vi "target.vi"   [LabVIEW 2020]
uses:
  <vilib>/rvi/interface/RandomDataEmulation/niFpgaRandomDataHandleErrors.vi
  matrix_matrix_multiply_FXP_16_4.vi
  <vilib>/rvi/DataTransferAndStorage/Container/XNode/niFpgaContainer.xnode
  <vilib>/rvi/interface/RandomDataEmulation/nirviRandomDataFpgaReadWriteTemplate.vi
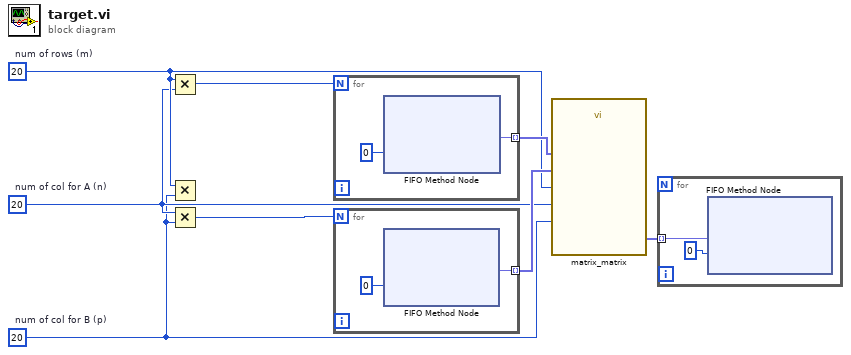
[diagram p0: block diagram]
diagram:
  w2 = 20  # num of col for B (p)
  w3 = 20  # num of col for A (n)
  w4 = 20  # num of rows (m)
  n1 = Multiply(x=w4, y=w3) -> (x*y=w8:i32)
  n2 = Multiply(x=w4, y=w2) -> ()  [unwired: 1 out]
  n3 = Multiply(x=w3, y=w2) -> (x*y=w7:i32)
  n4 = for {
    N: w8 -> [_]
    tunnel: [w10] -> w6 mode=indexing
    n5 = xnode ("FIFO Method Node")("Timeout"=0) -> ("Element"=w10:fxp<+/-,16,4>)  [unwired: 1 in, 2 out]
  }
  n6 = for {
    N: w7 -> [_]
    tunnel: [w11] -> w5 mode=indexing
    n7 = xnode ("FIFO Method Node")("Timeout"=0) -> ("Element"=w11:fxp<+/-,16,4>)  [unwired: 1 in, 2 out]
  }
  n8 = call-poly "matrix_matrix.vi"("p"=w2, "n"=w3, "m"=w4, "B"=w5, "A"=w6) -> ("C"=w1:fxp<+/-,16,4>[])  [unwired: 1 in]
  n9 = for {
    tunnel: w1 -> [w14] mode=indexing
    n10 = xnode ("FIFO Method Node")("Element"=w14, "Timeout"=0) -> ()  [unwired: 1 in, 2 out]
  }
